vi "Disable Custom Device.vi"(8 "error in (no error)":errorcluster, 11 "Ballard ARINC 429 ref":T1 format="%.0x") -> (0 "error out":errorcluster, 3 "Ballard ARINC 429 ref out":T1 format="%.0x")   [LabVIEW 2020, in "Ballard ARINC 429 Scripting.lvlib"]
doc: "Disables a Ballard ARINC 429 custom device."
uses:
  Ballard ARINC 429 Scripting.lvlib
  <vilib>/NI VeriStand/Custom Device API/Custom Device Item Ref.ctl
  NationalInstruments.VeriStand.SystemDefinitionAPI
  Constants.vi
  <vilib>/NI VeriStand/Custom Device API/Custom Device API.lvlib
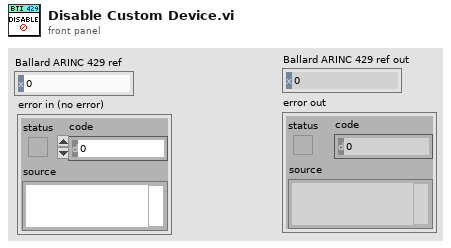
[diagram p1: front panel]
types:
  T1 = typedef "Custom Device API.lvlib/Custom Device Item Ref.ctl" = u64
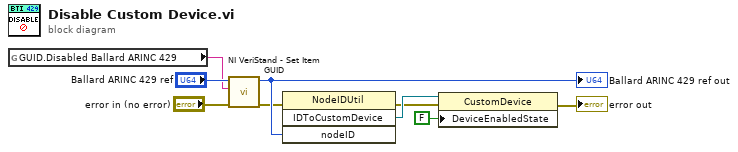
[diagram p0: block diagram]
diagram:
  n1 = global read "Constants.vi" "GUID.Disabled Ballard ARINC 429"() -> (w8:string)
  n2 = call <vilib>:"NI VeriStand - Set Item GUID.vi"("error in (no error)"="error in (no error)", "GUID"=w8, "Item Ref in"="Ballard ARINC 429 ref") -> ("error out"=w2:errorcluster, "Item Ref out"=w6:T1)  [unwired: 7 in]
  "Ballard ARINC 429 ref out" <- w6
  n3 = invoke class="NodeIDUtil" method="IDToCustomDevice"(error in=w2, "nodeID"=w6) -> (error out=w3:errorcluster, "IDToCustomDevice"=w5:refnum<k24>)  [unwired: 2 in, 2 out]
  n4 = property class="CustomDevice"(reference=w5, error in=w3, "DeviceEnabledState"=FALSE) -> (error out=→"error out":errorcluster)  [unwired: 1 out]
